vi "Read Application Config.vi"(8 "error in (no error)":errorcluster, 9 "Config Type In":variant, 10 "Section":string, 11 "Application in":refnum<data-value>) -> (0 "error out":errorcluster, 1 "Config Data out":variant, 3 "Application out":refnum<data-value>)   [LabVIEW 2015, in "Application.lvclass"]
uses:
  Application.lvclass
  Member Access/Read Path.vi
  <vilib>/Utility/config.llb/NI_LVConfig.lvlib
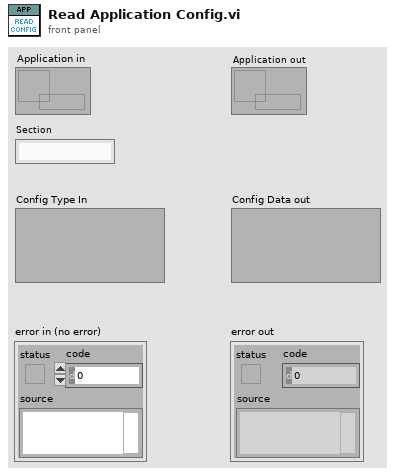
[diagram p1: front panel]
types:
  T1 = typedef "NI_LVConfig.lvlib/Config Data RefNum.ctl" = refnum<k1>
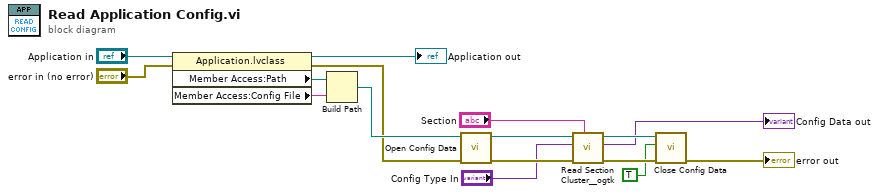
[diagram p0: block diagram]
diagram:
  n1 = property class="Application.lvclass"(reference="Application in", error in="error in (no error)") -> (reference out=→"Application out":refnum<data-value>, error out=w8:errorcluster, "Member Access:Path"=w15:path, "Member Access:Config File"=w16:string)
  n2 = Build Path(base path=w15, name or relative path=w16) -> (appended path=w14:path)
  n3 = call <vilib>:"Open Config Data.vi"("error in (no error)"=w8, "configuration file path"=w14) -> ("error out"=w12:errorcluster, "refnum"=w13:T1)  [unwired: 7 in, 1 out]
  n4 = call <userlib>:"Read Section Cluster__ogtk.vi"("section (optional)"="Section", "error in (no error)"=w12, "Section Formatted Cluster Type"="Config Type In", "refnum"=w13) -> ("error out"=w7:errorcluster, "Section Formatted Cluster"=→"Config Data out":variant, "dup refnum"=w6:T1)  [unwired: 3 in, 2 out]
  n5 = call <vilib>:"Close Config Data.vi"("error in (no error)"=w7, "write file if changed (T)"=TRUE, "refnum"=w6) -> ("error out"=→"error out":errorcluster)  [unwired: 7 in, 1 out]
